vi "F_TIMER.vi"(1 "Enum-Read/Write":T1) -> (0 "timer":u32)   [LabVIEW 2013]
uses:
  Control/Read&Write.ctl
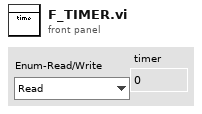
[diagram p1: front panel]
types:
  T1 = typedef "Read&Write.ctl" = enum16{"Read", "Write"}
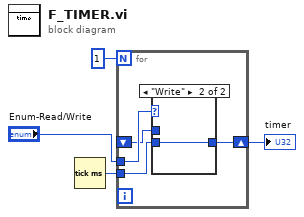
[diagram p0: block diagram]
diagram:
  n1 = Tick Count (ms)() -> (millisecond timer value=w3:u32)
  n2 = for {
    N: 1 -> [_]
    tunnel: "Enum-Read/Write" -> [w8]
    shift-right: [w7] -> w2
    shift-left: _ -> [w6]
    tunnel: w3 -> [w5]
    n3 = case shown="\"Write\"" w8 {
      tunnel: [w9 w10] -> w7
      tunnel: w6 -> [w9 _]
      tunnel: w5 -> [_ w10]
      frame "Read", Default {
      }
      frame "Write" {
      }
    }
  }
  "timer" <- w2
